vi "add tag.vi"(8 "error in":errorcluster, 10 "tag":refnum<class "data bus tag description.lvclass">, 11 "tag collection in":refnum<class "data bus tag collection.lvclass">) -> (0 "error out":errorcluster, 3 "tag collection out":refnum<class "data bus tag collection.lvclass">)   [LabVIEW 2013, in "data bus tag collection.lvclass"]
uses:
  data bus tag collection.lvclass
  tag/data bus tag description.lvclass
  data bus tag collection.lvclass/data bus tag collection.ctl
  tag/data bus tag description.lvclass/data bus tag description.ctl
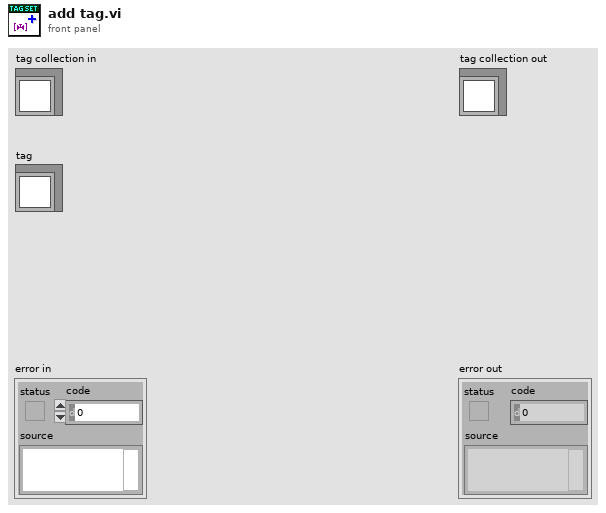
[diagram p1: front panel]
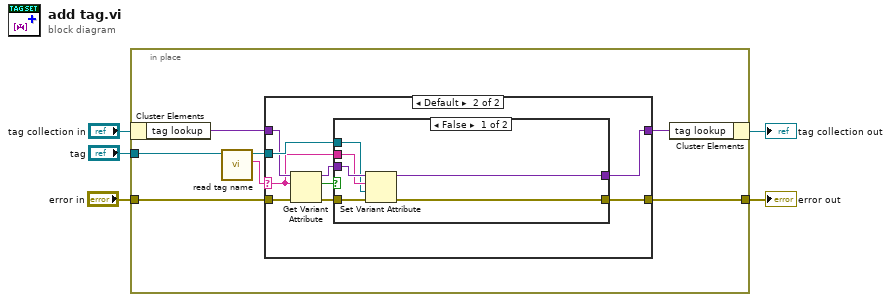
[diagram p0: block diagram]
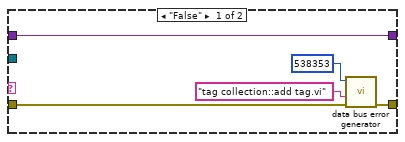
[diagram p2: hidden frame]
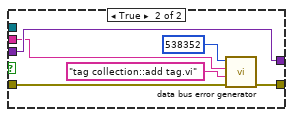
[diagram p3: hidden frame]
diagram:
  n1 = in-place {
    in-place-border: "error in" -> [w6]
    in-place-border: [w11] -> w2
    in-place-border: "tag" -> [w12]
    n2 = in-place-cluster #1("tag collection in") -> ("tag lookup"=w8:variant)
    n3 = call "read tag name.vi"("system tag in"=w12) -> ("name"=w7:string, "system tag out"=w9:refnum<class "data bus tag description.lvclass">)  [unwired: 8 in, 1 out]
    n4 = case shown="Default" w7 {
      selector: w7 -> [_ w21]
      tunnel: [w15 w26] -> w11
      tunnel: w6 -> [w14 w20]
      tunnel: w8 -> [w13 w23]
      tunnel: [w13 w25] -> w10
      tunnel: w9 -> [_ w24]
      frame "False" {
        n5 = call "data bus error generator.vi"("error in"=w14, "source"="tag collection::add tag.vi", "error code (0)"=538353) -> ("error out"=w15:errorcluster)  [unwired: 6 in]
      }
      frame Default {
        n6 = Get Variant Attribute(Variant=w23, name=w21, error in=w20) -> (duplicate Variant=w22:variant, found=w18:bool, error out=w19:errorcluster)  [unwired: 1 in, 1 out]
        n7 = case shown="False" w18 {
          tunnel: [w31 w36] -> w26
          tunnel: w19 -> [w32 w37]
          tunnel: w22 -> [w30 w38]
          tunnel: [w29 w38] -> w25
          tunnel: w24 -> [w27 _]
          tunnel: w21 -> [w28 w33]
          frame False {
            n8 = Set Variant Attribute(Variant=w30, name=w28, value=w27, error in=w32) -> (Variant out=w29:variant, error out=w31:errorcluster)  [unwired: 1 out]
          }
          frame True {
            n9 = call "data bus error generator.vi"("error in"=w37, "source"="tag collection::add tag.vi", "append error message"=w33, "error code (0)"=538352) -> ("error out"=w36:errorcluster)  [unwired: 5 in]
          }
        }
      }
    }
    n10 = in-place-cluster #1("tag lookup"=w10) -> (→"tag collection out":refnum<class "data bus tag collection.lvclass">)
  }
  "error out" <- w2
